vi "Grid_Checks.vi"(10 "Settings":T1={"Drift Correction Settings"={"Drift Correction every"=80, "Drift correction Pixels"=256, "Channel index (0-23)"=0, "MaxImagesBack"=2, "Threshold"=2, "Increment"=8, "max applied Drift Correction"=20, "Correct Drift"=TRUE, "Correlate"=0, "Correct z drift"=FALSE, "zdrift \nDuration (s)"=0.0}, "Spectroscopy Setting"={"Imaging Current"=1e-11, "ref Current"=7e-11, "tip Speed (m/s)"=2e-09, "Imaging Bias"=0.02, "ref Bias"=-0.1, "preSTS delay [ms]"=500, "STS z offset"=2e-10, "during Spec Bias (V)"=-0.1, "trigger1 < Hz"=0.0, "trigger 2 >Hz"=0.0, "autoStop"=FALSE, "Spectroscopy"=0, "PLL ON/OFF"=TRUE, "readjust setpoint every "=1, "z Reference"=FALSE, "Lock In"=TRUE}, "Misc"={"File name"="symmetric_node_zOff=200p", "Email when finished"="cornelius.krull@monash.edu,Dhaneesh.Gopalakrishnan@monash.edu,marina.castelli@monash.edu"}, "Grid Settings"={"type"=1, "type order"=1, "X pixel"=0, "Y pixel"=0, "Grid_Parms"={"center X (m)"=0.0, "center Y (m)"=0.0, "width (m)"=0.0, "height (m)"=0.0, "angle (deg)"=0.0}}} {"Grid Settings"."type order" items=["Grid", "Random", "Adam7"]; "Grid Settings"."type" items=["Line", "Grid"]; "Spectroscopy Setting"."Spectroscopy" items=["Bias", "zSpec"]; "Spectroscopy Setting"."trigger 2 >Hz" format="%#_6p"; "Spectroscopy Setting"."trigger1 < Hz" format="%#_6p"; "Spectroscopy Setting"."during Spec Bias (V)" format="%#_5p"; "Spectroscopy Setting"."STS z offset" format="%#_6p"; "Spectroscopy Setting"."ref Bias" format="%#_6p"; "Spectroscopy Setting"."Imaging Bias" format="%#_6p"; "Spectroscopy Setting"."tip Speed (m/s)" format="%.2p"; "Spectroscopy Setting"."ref Current" format="%#_6p"; "Spectroscopy Setting"."Imaging Current" format="%#_6p"; "Drift Correction Settings"."Correlate" items=["first Frame", "successive Frames"]; "Drift Correction Settings"."max applied Drift Correction" min=1 max=100 step=1 format="%.0p"; "Drift Correction Settings"."Threshold" min=1 step=1; "Drift Correction Settings"."Channel index (0-23)" items=["Current"=0, "Z (m)"=14]}) -> (2 "Settings out":T1={"Drift Correction Settings"={"Drift Correction every"=80, "Drift correction Pixels"=256, "Channel index (0-23)"=0, "MaxImagesBack"=2, "Threshold"=2, "Increment"=8, "max applied Drift Correction"=20, "Correct Drift"=TRUE, "Correlate"=0, "Correct z drift"=FALSE, "zdrift \nDuration (s)"=0.0}, "Spectroscopy Setting"={"Imaging Current"=1e-11, "ref Current"=7e-11, "tip Speed (m/s)"=2e-09, "Imaging Bias"=0.02, "ref Bias"=-0.1, "preSTS delay [ms]"=500, "STS z offset"=2e-10, "during Spec Bias (V)"=-0.1, "trigger1 < Hz"=0.0, "trigger 2 >Hz"=0.0, "autoStop"=FALSE, "Spectroscopy"=0, "PLL ON/OFF"=TRUE, "readjust setpoint every "=1, "z Reference"=FALSE, "Lock In"=TRUE}, "Misc"={"File name"="symmetric_node_zOff=200p", "Email when finished"="cornelius.krull@monash.edu,Dhaneesh.Gopalakrishnan@monash.edu,marina.castelli@monash.edu"}, "Grid Settings"={"type"=1, "type order"=1, "X pixel"=0, "Y pixel"=0, "Grid_Parms"={"center X (m)"=0.0, "center Y (m)"=0.0, "width (m)"=0.0, "height (m)"=0.0, "angle (deg)"=0.0}}} {"Grid Settings"."type order" items=["Grid", "Random", "Adam7"]; "Grid Settings"."type" items=["Line", "Grid"]; "Spectroscopy Setting"."Spectroscopy" items=["Bias", "zSpec"]; "Spectroscopy Setting"."trigger 2 >Hz" format="%#_6p"; "Spectroscopy Setting"."trigger1 < Hz" format="%#_6p"; "Spectroscopy Setting"."during Spec Bias (V)" format="%#_5p"; "Spectroscopy Setting"."STS z offset" format="%#_6p"; "Spectroscopy Setting"."ref Bias" format="%#_6p"; "Spectroscopy Setting"."Imaging Bias" format="%#_6p"; "Spectroscopy Setting"."tip Speed (m/s)" format="%.2p"; "Spectroscopy Setting"."ref Current" format="%#_6p"; "Spectroscopy Setting"."Imaging Current" format="%#_6p"; "Drift Correction Settings"."Correlate" items=["first Frame", "successive Frames"]; "Drift Correction Settings"."max applied Drift Correction" min=1 max=100 step=1 format="%.0p"; "Drift Correction Settings"."Threshold" min=1 step=1; "Drift Correction Settings"."Channel index (0-23)" items=["Current"=0, "Z (m)"=14]})   [LabVIEW 2021]
panel:
  # "z Spectroscopy"
  # "GRID points"
  # "Increase this if no Drift was detected for \na certain number of images"
  # "% of image size"
  # "z Spectroscopy"
  # "GRID points"
  # "Increase this if no Drift was detected for \na certain number of images"
  # "% of image size"
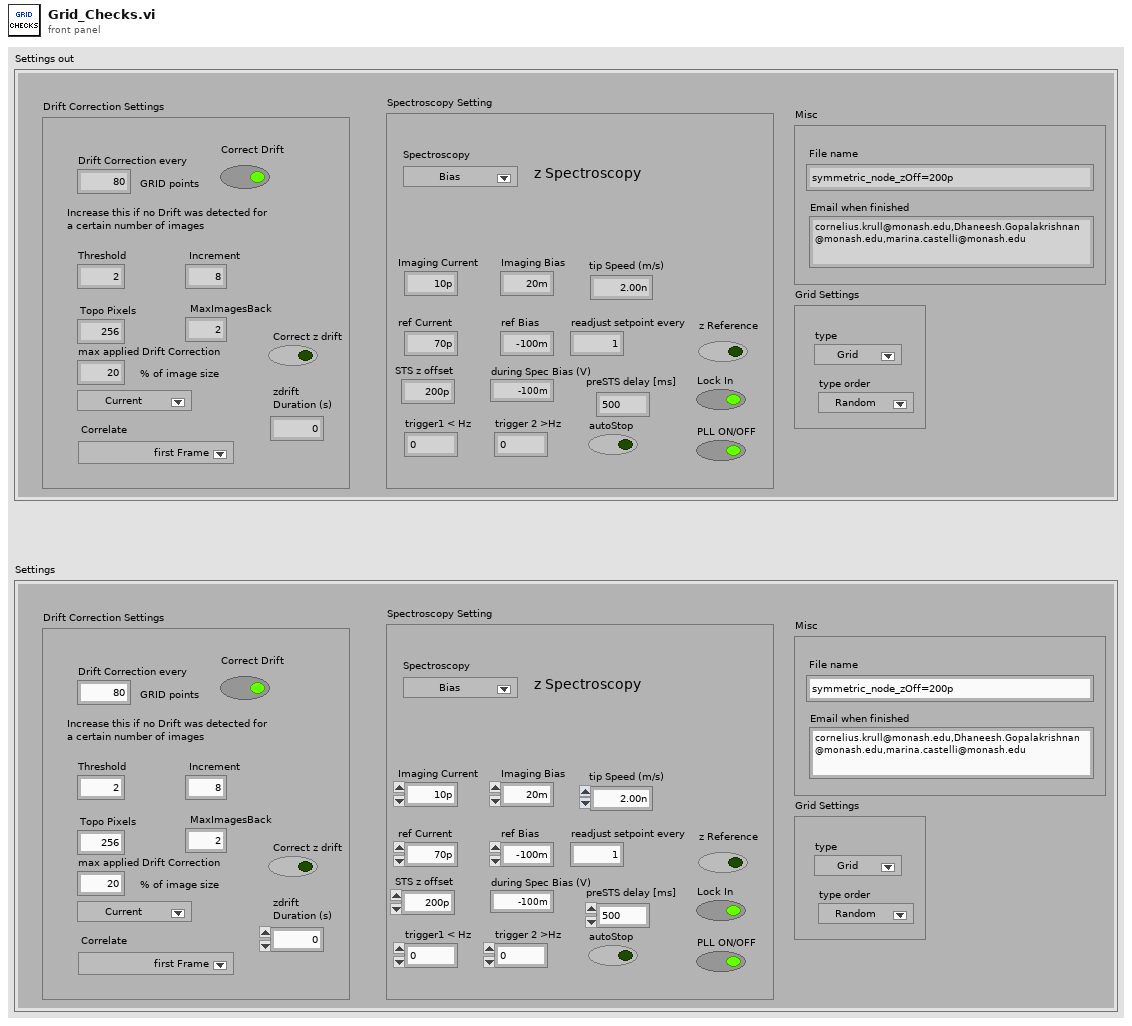
[diagram p1: front panel]
types:
  T1 = cluster{"Drift Correction Settings":cluster{"Drift Correction every":i32, "Drift correction Pixels":i32, "Channel index (0-23)":u8, "MaxImagesBack":i32, "Threshold":i32, "Increment":i32, "max applied Drift Correction":i32, "Correct Drift":bool, "Correlate":u16, "Correct z drift":bool, "zdrift \nDuration (s)":dbl}, "Spectroscopy Setting":cluster{"Imaging Current":dbl, "ref Current":dbl, "tip Speed (m/s)":sgl, "Imaging Bias":dbl, "ref Bias":dbl, "preSTS delay [ms]":u32, "STS z offset":dbl, "during Spec Bias (V)":sgl, "trigger1 < Hz":sgl, "trigger 2 >Hz":sgl, "autoStop":bool, "Spectroscopy":u16, "PLL ON/OFF":bool, "readjust setpoint every ":i32, "z Reference":bool, "Lock In":bool}, "Misc":cluster{"File name":string, "Email when finished":string}, "Grid Settings":cluster{"type":u16, "type order":u16, "X pixel":i32, "Y pixel":i32, "Grid_Parms":cluster{"center X (m)":sgl, "center Y (m)":sgl, "width (m)":sgl, "height (m)":sgl, "angle (deg)":sgl}}}
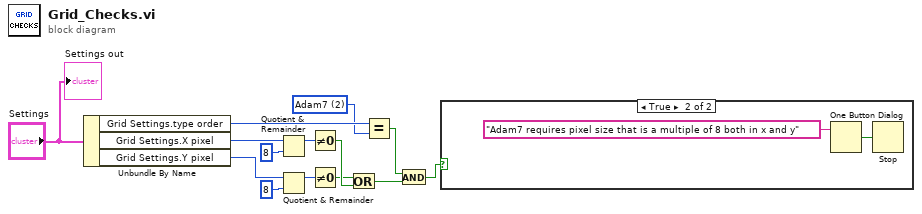
[diagram p0: block diagram]
diagram:
  w1 = u16 2 items=["Grid", "Random", "Adam7"] ("type order")
  n1 = Unbundle By Name("Settings") -> ("Grid Settings.type order"=w14:u16, "Grid Settings.X pixel"=w11:i32, "Grid Settings.Y pixel"=w12:i32)
  n2 = Quotient & Remainder(x=w11, y=8) -> (x-y*floor(x/y)=w7:i32)  [unwired: 1 out]
  n3 = Quotient & Remainder(x=w12, y=8) -> (x-y*floor(x/y)=w8:i32)  [unwired: 1 out]
  n4 = Not Equal To 0?(x=w7) -> (x != 0?=w4:bool)
  n5 = Not Equal To 0?(x=w8) -> (x != 0?=w3:bool)
  n6 = Or(x=w3, y=w4) -> (x .or. y?=w2:bool)
  n7 = Equal?(x=w14, y=w1) -> (x = y?=w5:bool)
  n8 = And(x=w5, y=w2) -> (x .and. y?=w6:bool)
  n9 = case shown="True" w6 {
    frame False {
    }
    frame True {
      n10 = One Button Dialog(message="Adam7 requires pixel size that is a multiple of 8 both in x and y") -> (true=w15:bool)  [unwired: 1 in]
      n11 = Stop(stop? (T)=w15) -> ()
    }
  }
  "Settings out" <- "Settings"
